vi "Duplicate.vi"(8 "error in":errorcluster, 10 "parameters":variant, 11 "SwitchACIR Channel":refnum<class "SwitchACIR Channel.lvclass">) -> (0 "error out":errorcluster, 3 "SwitchACIR Channel copy":refnum<class "SwitchACIR Channel.lvclass">)   [LabVIEW 2025, in "SwitchACIR Channel.lvclass"]
doc: "Implements the specific behavior of a node when it is being duplicated\nCan be used to change the name of the new node for example adding Copy to it. \nCopyright 2017 National Instruments Corporation\n\nLicensed under the Apache License, Version 2.0 (the \"License\"); you may not use this file except in compliance with the License. You may obtain a copy of the License at http://www.apache.org/licenses/LICENSE-2.0\nUnless required by applicable law or agreed to in writing, software distributed under the License is distributed on an \"AS IS\" BASIS, WITHOUT WARRANTIES OR CONDITIONS OF ANY KIND, either express or implied. See the License for the specific language governing permissions and limitations under the License."
uses:
  SwitchACIR Channel.lvclass
  SwitchACIR Channel.lvclass/SwitchACIR Channel.ctl
  SwitchACIR Channel configuration/SwitchACIR Channel configuration.lvclass
  C:/Users/Public/Documents/Sandia National Labs/TSS Plugin/Abstract Engine.lvlibp/Channel configuration/Channel configuration.lvclass
  Users/Public/Documents/Sandia National Labs/TSS Plugin/Abstract Engine.lvlibp/Channel configuration/Read Channel Setting.vi
  Users/Public/Documents/Sandia National Labs/TSS Plugin/Abstract Engine.lvlibp/Channel configuration/Write Channel Setting.vi
  Users/Public/Documents/Sandia National Labs/TSS Plugin/Abstract Engine.lvlibp/Abstract Channel/Abstract Channel.lvclass
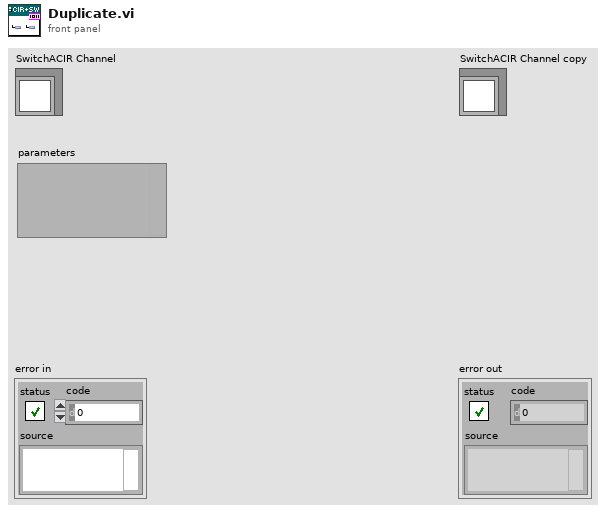
[diagram p1: front panel]
types:
  T1 = typedef "Abstract Engine.lvlibp/Channel configuration.lvclass/Default Channel.ctl" = cluster{"Address":string, "SW Alias":string, "Enabled":bool, "Type":string, "Description":string}
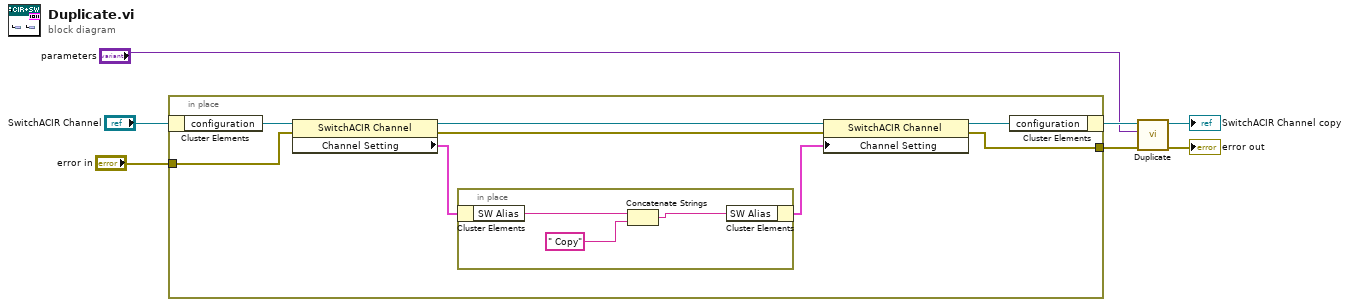
[diagram p0: block diagram]
diagram:
  n1 = in-place {
    in-place-border: "error in" -> [w12]
    in-place-border: [w8] -> w1
    n2 = in-place-cluster #1("SwitchACIR Channel") -> ("configuration"=w15:refnum<class "SwitchACIR Channel configuration.lvclass">)
    n3 = property class="SwitchACIR Channel"(reference=w15, error in=w12) -> (reference out=w13:refnum<class "SwitchACIR Channel configuration.lvclass">, error out=w9:errorcluster, "Channel Setting"=w11:T1)
    n4 = in-place {
      n5 = in-place-cluster #2(w11) -> ("SW Alias"=w18:string)
      n6 = Concatenate Strings(w18, " Copy") -> (w17:string)
      n7 = in-place-cluster #2("SW Alias"=w17) -> (w10:T1)
    }
    n8 = property class="SwitchACIR Channel"(reference=w13, error in=w9, "Channel Setting"=w10) -> (reference out=w14:refnum<class "SwitchACIR Channel configuration.lvclass">, error out=w8:errorcluster)
    n9 = in-place-cluster #1("configuration"=w14) -> (w7:refnum<class "SwitchACIR Channel.lvclass">)
  }
  n10 = call-parent "Duplicate.vi"("error in"=w1, "parameters"="parameters", "CEF_Serialize node in"=w7) -> ("error out"=→"error out":errorcluster, "CEF_Serialize node out"=→"SwitchACIR Channel copy":refnum<class "SwitchACIR Channel.lvclass">)  [unwired: 7 in]
